vi "test_main.vi"() -> ()   [LabVIEW 2023, in "Easy.SequenceManager.Test.lvlib"]
uses:
  Easy.SequenceManager.Test.lvlib
panel:
  in  "error in (no error)":errorcluster
  out "error out":errorcluster
  # "Locals"
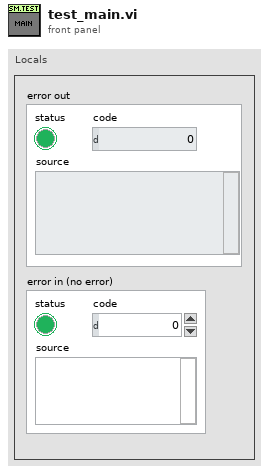
[diagram p1: front panel]
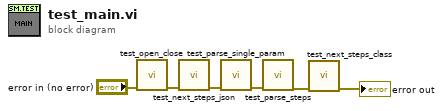
[diagram p0: block diagram]
diagram:
  n1 = call "test_open_close.vi"("error in (no error)"="error in (no error)") -> ("error out"=w6:errorcluster)  [unwired: 10 in]
  n2 = call "test_next_steps_json.vi"("error in (no error)"=w6) -> ("error out"=w5:errorcluster)  [unwired: 10 in]
  n3 = call "test_parse_single_param.vi"("error out 2"=w5) -> ("error out"=w4:errorcluster)  [unwired: 10 in]
  n4 = call "test_parse_steps.vi"("error in"=w4) -> ("error out"=w2:errorcluster)  [unwired: 10 in]
  n5 = call "test_next_steps_class.vi"("error in (no error)"=w2) -> ("error out"=→"error out":errorcluster)  [unwired: 10 in]
